vi "Write Offline Log.vi"(8 "error in (no error)":errorcluster, 10 "Offline Log":string, 11 "Log.Litho in":refnum<class "Log.Litho.lvclass">) -> (0 "error out":errorcluster, 3 "Log.Litho out":refnum<class "Log.Litho.lvclass">)   [LabVIEW 2019, in "Log.Litho.lvclass"]
uses:
  Log.Litho.lvclass
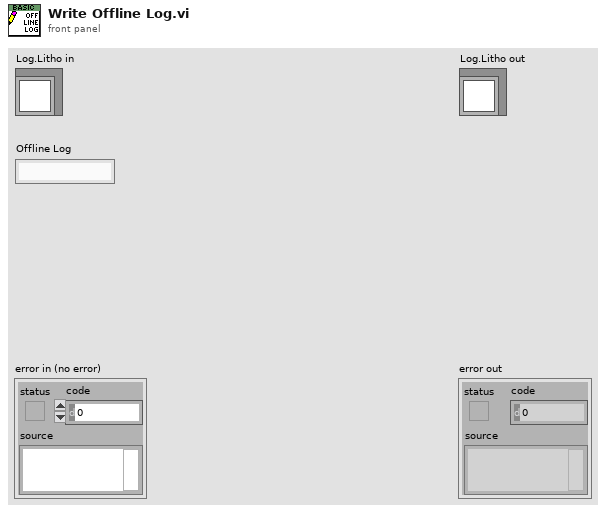
[diagram p1: front panel]
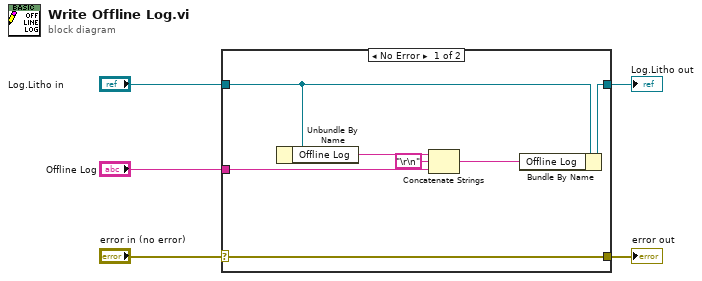
[diagram p0: block diagram]
diagram:
  n1 = case shown="No Error" "error in (no error)" {
    selector: "error in (no error)" -> [w12 w13]
    tunnel: [w12 w13] -> w4
    tunnel: [w11 w14] -> w2
    tunnel: "Log.Litho in" -> [w9 w14]
    tunnel: "Offline Log" -> [w6 _]
    frame No Error {
      n2 = Unbundle By Name(w9) -> ("Offline Log"=w8:string)
      n3 = Concatenate Strings(w8, "\r\n", w6) -> (w7:string)
      n4 = Bundle By Name(cluster=w9, "Offline Log"=w7) -> (w11:refnum<class "Log.Litho.lvclass">)
    }
    frame Error {
    }
  }
  "error out" <- w4
  "Log.Litho out" <- w2
